vi "GetMatchData.vi"(7 "Update?":bool, 8 "MatchData":string) -> (3 "MatchDataOut":string)   [LabVIEW 2017]
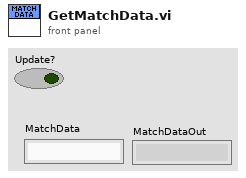
[diagram p1: front panel]
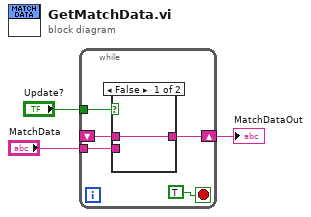
[diagram p0: block diagram]
diagram:
  n1 = while {
    shift-right: [w7] -> w1
    shift-left: _ -> [w8]
    tunnel: "MatchData" -> [w6]
    tunnel: "Update?" -> [w5]
    stop <- TRUE stop-if-true
    n2 = case shown="False" w5 {
      tunnel: w8 -> [w9 _]
      tunnel: [w9 w10] -> w7
      tunnel: w6 -> [_ w10]
      frame False {
      }
      frame True {
      }
    }
  }
  "MatchDataOut" <- w1
